vi "IntegerRanges.vi"() -> ()   [LabVIEW 2019]
panel:
  in  "I64":i64
  in  "u64":u64
  in  "I32":i32
  in  "u32":u32
  in  "I16":i16
  in  "u16":u16
  in  "I8":i8
  in  "u8":u8
  # "0-65535"
  # "-32768 - 32767"
  # "0 - 4294967295"
  # "-2147483648 - 2147483647"
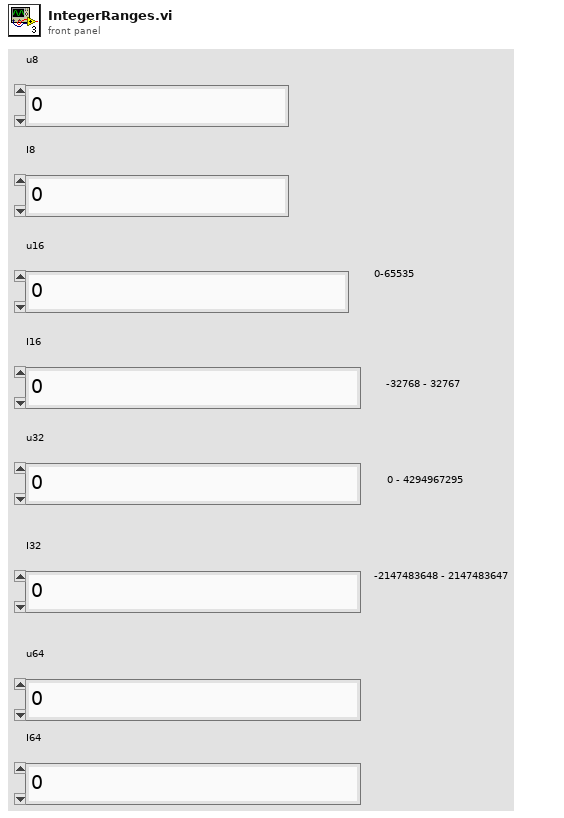
[diagram p1: front panel]
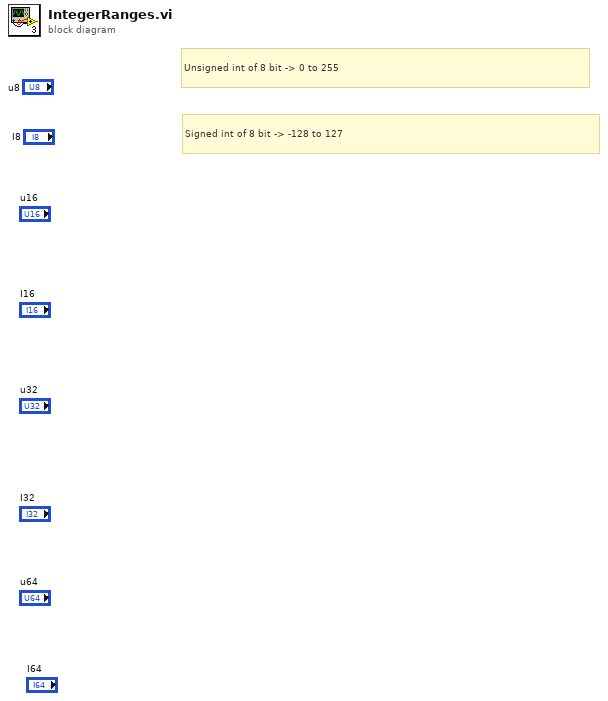
[diagram p0: block diagram]
diagram:
  # "Signed int of 8 bit -> -128 to 127"
  # "Unsigned int of 8 bit -> 0 to 255"
